vi "createFakeImage.vi"(8 "error in":errorcluster, 11 "FPGA VI Reference":T1) -> (0 "error out":errorcluster, 1 "ready for data":bool, 2 "fake 2 ch im":u32[](array[numeric]), 3 "FPGA VI Reference Out":T1)   [LabVIEW 2010]
uses:
  FPGA_ref.ctl
  <vilib>/rvi/interface/nirviMethod/nirviMethod.xnode
  <vilib>/rvi/interface/common/niFpgaNodeNameForErrorReporting.ctl
  <vilib>/rvi/errors/niLvFpgaWhatHappensToTopLevelVI.ctl
  <vilib>/rvi/interface/nirviReadWriteControl/nirviReadWriteControl.xnode
  <vilib>/Utility/error.llb/Error Cluster From Error Code.vi
  <vilib>/rvi/errors/niLvFpgaAdjustHostInterfaceError.vi
  NiFpgaLv.dll
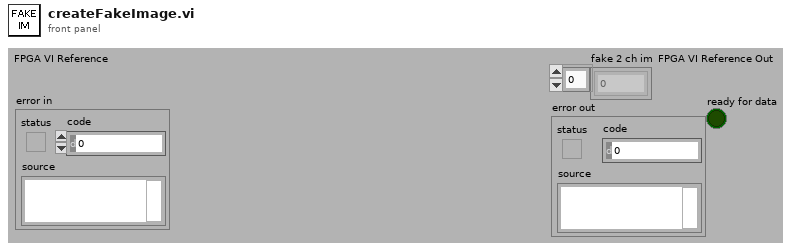
[diagram p1: front panel]
types:
  T1 = typedef "FPGA_ref.ctl" = refnum<k20>
  T2 = cluster{"x amplitude":u16, "x resolution (pixels)":u16, "x offset fly-forward (iterations)":u16, "x offset fly-back (iterations)":u16, "y resolution (nr. of lines)":u16, "y step size":u16, "iterations per pixel":u16, "number of frames":i32, "y offset (pixels)":u16, "number of y-brake lines  (before y-fly-back)":u16, "number y-brake lines (after y-fly-back)":u16, "number of y-fly-back steps":u16, "lines per z step":u16, "number of z/intensity tuples":u16, "number of repetitions (volumes or planes)":i32, "z step size derived":u16, "choose the beginning of z scan":bool, "number of frames (settings)":i32, "FPGA trajectory?":bool, "Pockels cell voltage (bits)":i16, "Vy min(bits)":i16, "Vz min(bits)":i16}
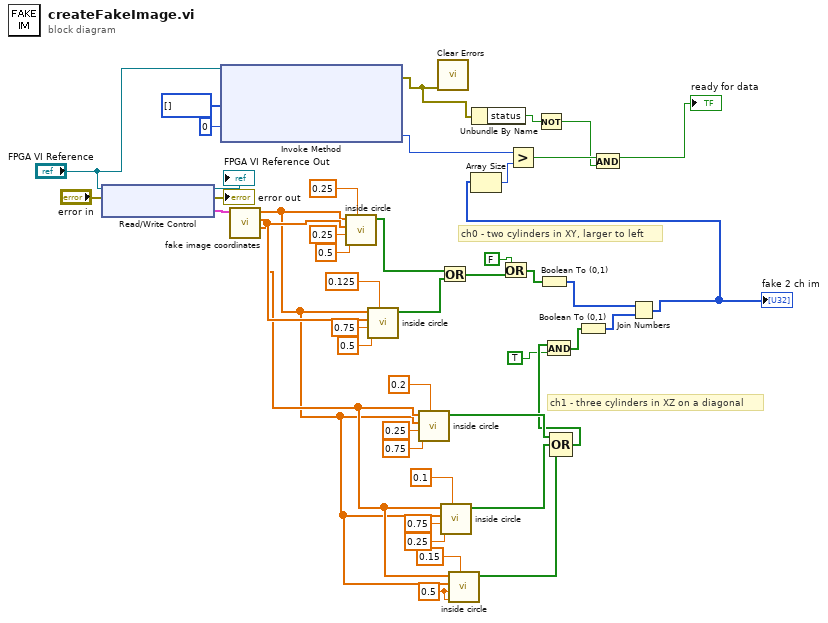
[diagram p0: block diagram]
diagram:
  w26 = 0.5 ("xc")
  # "ch1 - three cylinders in XZ on a diagonal"
  # "ch0 - two cylinders in XY, larger to left"
  n1 = xnode "Read/Write Control"("FPGA VI Reference In"="FPGA VI Reference", "error in"="error in") -> ("FPGA VI Reference Out"=→"FPGA VI Reference Out":T1, "error out"=→"error out":errorcluster, "scan specification"=w44:T2)
  n2 = xnode "Invoke Method"("FPGA VI Reference In"="FPGA VI Reference", "Data"=u32[] [], "Timeout (ms)"=0) -> ("error out"=w4:errorcluster, "Empty Elements Remaining"=w9:u32)  [unwired: 1 in, 1 out]
  n3 = call "fake image coordinates.vi"("scan specification"=w44) -> ("zcoords"=w28:dbl[], "ycoords"=w37:dbl[], "xcoords"=w27:dbl[])  [unwired: 8 in]
  n4 = call "inside circle.vi"("r"=0.25, "yc"=0.5, "xc"=0.25, "ycoords"=w37, "xcoords"=w27) -> ("inside circle"=w36:bool[])  [unwired: 6 in]
  n5 = call "inside circle.vi"("r"=0.125, "yc"=0.5, "xc"=0.75, "ycoords"=w37, "xcoords"=w27) -> ("inside circle"=w35:bool[])  [unwired: 6 in]
  n6 = call "inside circle.vi"("r"=0.2, "yc"=0.75, "xc"=0.25, "ycoords"=w27, "xcoords"=w28) -> ("inside circle"=w24:bool[])  [unwired: 6 in]
  n7 = call <vilib>:"Clear Errors.vi"("error in (no error)"=w4) -> ()  [unwired: 6 in, 1 out]
  n8 = Or(x=w36, y=w35) -> (x .or. y?=w21:bool[])
  n9 = call "inside circle.vi"("r"=0.1, "yc"=0.25, "xc"=0.75, "ycoords"=w27, "xcoords"=w28) -> ("inside circle"=w23:bool[])  [unwired: 6 in]
  n10 = call "inside circle.vi"("r"=0.15, "yc"=w26, "xc"=w26, "ycoords"=w27, "xcoords"=w28) -> ("inside circle"=w22:bool[])  [unwired: 6 in]
  n11 = Unbundle By Name(w4) -> ("status"=w3:bool)
  n12 = Or(x=FALSE, y=w21) -> (x .or. y?=w15:bool[])
  n13 = Not(x=w3) -> (.not. x?=w1:bool)
  n14 = Boolean To (0,1)(Boolean=w15) -> (0, 1=w13:i16[])
  n15 = Compound Arithmetic op=OR(w24, w23, w22) -> (w20:bool[])
  n16 = And(x=w20, y=TRUE) -> (x .and. y?=w14:bool[])
  n17 = Boolean To (0,1)(Boolean=w14) -> (0, 1=w12:i16[])
  n18 = Join Numbers(hi=w13, lo=w12) -> ((hi.lo)=w8:u32[])
  "fake 2 ch im" <- w8
  n19 = Array Size(array=w8) -> (size(s)=w7:i32)
  n20 = Greater?(x=w9, y=w7) -> (0:w6:bool)
  n21 = And(x=w6, y=w1) -> (x .and. y?=→"ready for data":bool)
